vi "myCommClose_visa.vi"(6 "是否存在DSP":bool, 8 "错误输入（无错误）":errorcluster, 11 "VISA资源名称":refnum<visa-resource-name>) -> (1 "通信关机结果":string)   [LabVIEW 2024]
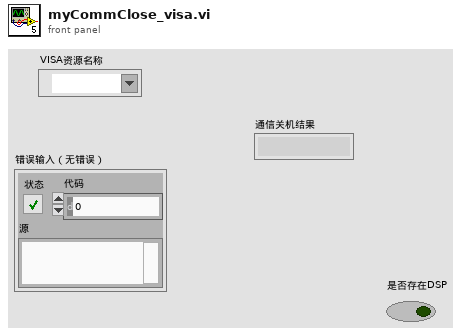
[diagram p1: front panel]
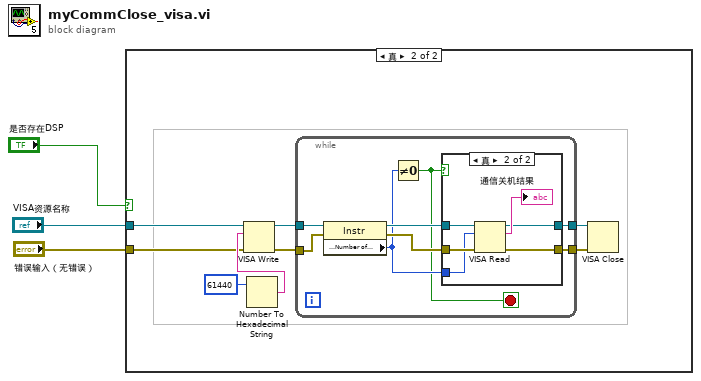
[diagram p0: block diagram]
diagram:
  n1 = case shown="真" "是否存在DSP" {
    tunnel: "VISA资源名称" -> [_ w5]
    tunnel: "错误输入（无错误）" -> [_ w4]
    frame False {
    }
    frame True {
      n2 = Number To Hexadecimal String(2:u16 61440) -> (0:w9:string)  [unwired: 1 in]
      n3 = VISA Write(VISA resource name=w5, write buffer=w9, error in (no error)=w4) -> (VISA resource name out=w11:refnum<visa-resource-name>, error out=w10:errorcluster)  [unwired: 1 out]
      n4 = while {
        tunnel: w11 -> [w19]
        tunnel: w10 -> [w12]
        tunnel: [w14] -> w6
        tunnel: [w13] -> w7
        stop <- w15 stop-if-true
        n5 = property class="Instr"(reference=w19, error in=w12) -> (reference out=w18:refnum<visa-resource-name>, error out=w17:errorcluster, "Serial Settings:Number of Bytes at Serial Port"=w16:u32)
        n6 = Not Equal To 0?(x=w16) -> (x != 0?=w15:bool)
        n7 = case shown="真" w15 {
          tunnel: w18 -> [w21 w26]
          tunnel: w17 -> [w20 w27]
          tunnel: w16 -> [_ w25]
          tunnel: [w20 w23] -> w14
          tunnel: [w21 w22] -> w13
          frame False {
          }
          frame True {
            n8 = VISA Read(VISA resource name=w26, byte count=w25, error in (no error)=w27) -> (VISA resource name out=w22:refnum<visa-resource-name>, read buffer=→"通信关机结果":string, error out=w23:errorcluster)  [unwired: 1 out]
          }
        }
      }
      n9 = VISA Close(VISA resource name=w7, error in (no error)=w6) -> ()  [unwired: 1 out]
    }
  }
